vi "Remove Image.vi"(0 "Image Ref":T1, 11 "Error In":errorcluster) -> (15 "Error Out":errorcluster)   [LabVIEW 2020]
uses:
  <vilib>/vision/Image Controls.llb/IMAQ Image.ctl
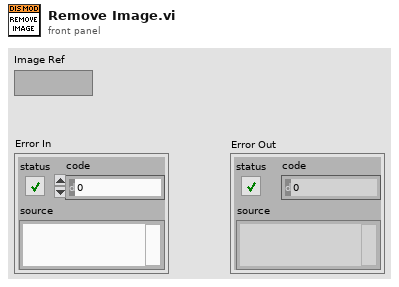
[diagram p1: front panel]
types:
  T1 = typedef "IMAQ Image.ctl" = refnum<image>
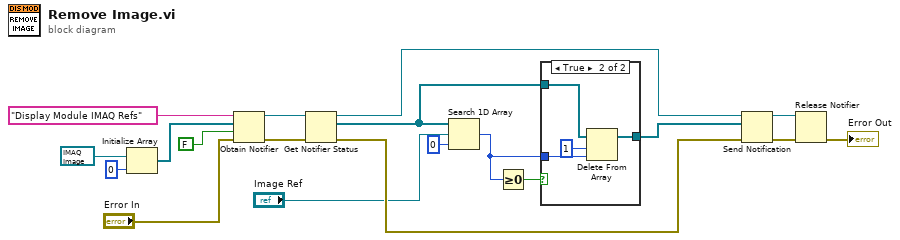
[diagram p0: block diagram]
diagram:
  n1 = Initialize Array(T1 refnum ("New Image"), 0 ("dimension size")) -> (w15:T1[])
  n2 = Obtain Notifier(name (unnamed)="Display Module IMAQ Refs", notification data type=w15, create if not found? (T)=FALSE, error in (no error)="Error In") -> (notifier out=w6:refnum<notifier>, error out=w5:errorcluster)  [unwired: 1 out]
  n3 = Get Notifier Status(notifier=w6, error in (no error)=w5) -> (notifier out=w13:refnum<notifier>, current notification=w14:T1[], error out=w12:errorcluster)  [unwired: 2 out]
  n4 = Search 1D Array(1D array=w14, element="Image Ref", start index (0)=0) -> (index of element=w2:i32)
  n5 = Greater Or Equal To 0?(x=w2) -> (x >= 0?=w3:bool)
  n6 = case shown="True" w3 {
    tunnel: w2 -> [_ w23]
    tunnel: w14 -> [w20 w22]
    tunnel: [w20 w21] -> w11
    frame False {
    }
    frame True {
      n7 = Delete From Array(array=w22, length=1, index=w23) -> (array with subset deleted=w21:T1[])  [unwired: 1 out]
    }
  }
  n8 = Send Notification(notification=w11, notifier=w13, error in (no error)=w12) -> (notifier out=w9:refnum<notifier>, error out=w8:errorcluster)
  n9 = Release Notifier(notifier=w9, error in (no error)=w8) -> (error out=→"Error Out":errorcluster)  [unwired: 1 in, 2 out]
